vi "save ROI overlay for arbitrary line scan.vi"(11 "ROI Descriptor":T1 {"Contours"."Type" items=["No Selection", "Point", "Line", "Rectangle", "Oval", "Polygon", "Freehand Region", "Annulus", "Unused2", "Unused3", "Broken Line", "Freehand Line", "Rotated Rectangle"]}) -> ()   [LabVIEW 2017]
doc: "SciScan 1.2 160622"
uses:
  GFG/GFGImageRefsGet.vi
  GFG/GFGDisplayRefsGet.vi
  <vilib>/Utility/file.llb/Write To Spreadsheet File (I64).vi
  GFG/GFG library.lvlib
  <vilib>/vision/NI_Vision_Development_Module.lvlib
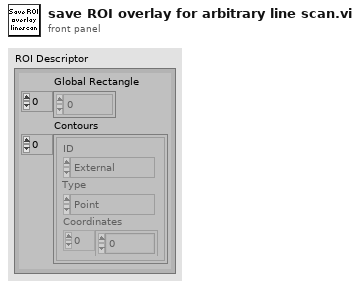
[diagram p1: front panel]
types:
  T1 = typedef "ROI Descriptor" = cluster{"Global Rectangle":i32[], "Contours":cluster{"ID":enum32{"External", "Internal"}, "Type":u32, "Coordinates":i32[]}[]}
  T2 = typedef "Image Type" = u32
  T3 = cluster{"Left":i32, "Top":i32, "Right":i32, "Bottom":i32}
  T4 = typedef "IMAQ Image.ctl" = refnum<image>
  T5 = cluster{"Channel 1 small":T4, "Channel 2 small":T4, "Channel 3 small":T4, "Channel 4 small":T4, "Channel 1 large":T4, "Channel 2 large":T4, "Channel 3 large":T4, "Channel 4 large":T4, "RGB overlay":T4, "ROI Image display":T4, "arb line scan display":T4, "Channel 5 large":T4}
  T6 = cluster{"Channel 1 small":refnum<vi>, "Channel 2 small":refnum<vi>, "Channel 3 small":refnum<vi>, "Channel 4 small":refnum<vi>, "Channel 1 large":refnum<vi>, "Channel 2 large":refnum<vi>, "Channel 3 large":refnum<vi>, "Channel 4 large":refnum<vi>, "RGB overlay":refnum<vi>, "ROI Image display":refnum<vi>, "arb line scan display":refnum<vi>, "Channel 5 large":refnum<vi>}
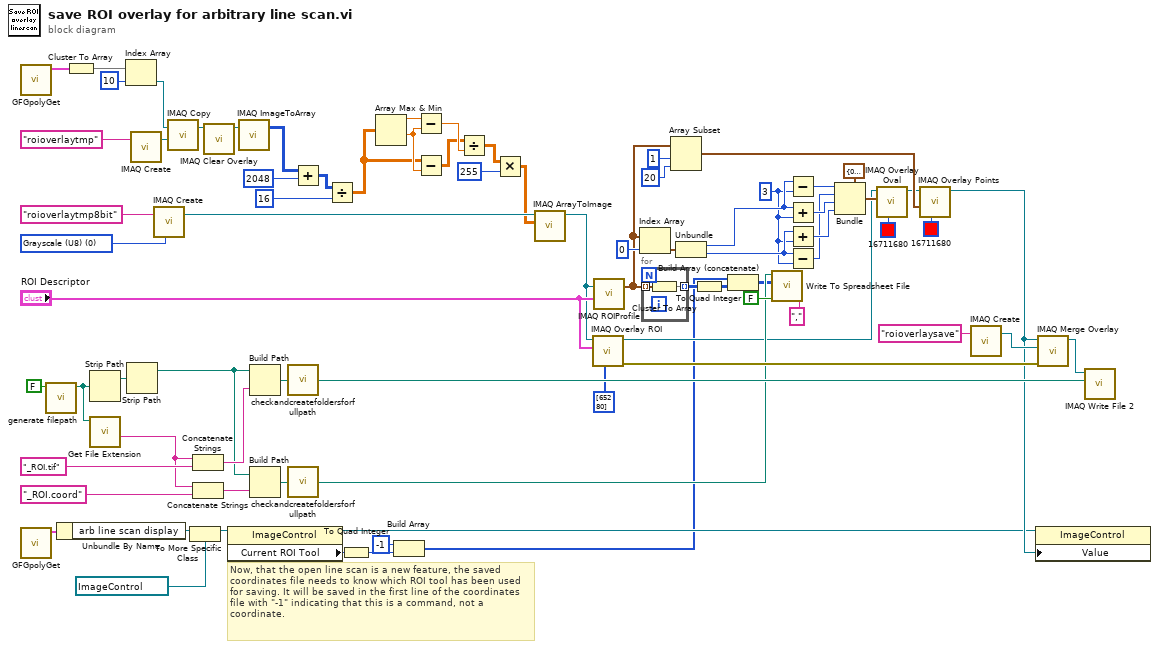
[diagram p0: block diagram]
diagram:
  w29 = T2 0 items=["Grayscale (U8)", "Grayscale (I16)", "Grayscale (SGL)", "Complex (CSG)", "RGB (U32)", "HSL (U32)", "RGB (U64)", "Grayscale (U16)"] ("Image Type")
  w11 = 3 ("y")
  # "Now, that the open line scan is a new feature, the saved coordinates file needs to know which ROI tool has been used for saving. It will be saved in the first line of the coordinates file with \"-1\" indicating that this is a command, not a coordinate."
  n1 = call-poly "GFGpolyGet.vi"() -> ("Image Refs Out"=w73:T5)  [unwired: 10 in, 1 out]
  n2 = call-poly "GFGpolyGet.vi"() -> ("DisplayRefsOut(generic class)"=w37:T6)  [unwired: 10 in, 1 out]
  n3 = call "generate filepath.vi"("set file.path GFG (default: T)"=FALSE) -> ("path"=w72:path)  [unwired: 10 in]
  n4 = Unbundle By Name(w37) -> ("arb line scan display"=w36:refnum<vi>)
  n5 = Cluster To Array(cluster=w73) -> (array=w75:T4[])
  n6 = Strip Path(path=w72) -> (stripped path=w68:path)  [unwired: 1 out]
  n7 = call <vilib>:"Get File Extension.vi"("file"=w72) -> ("filename without extension"=w63:string)  [unwired: 6 in, 4 out]
  n8 = Index Array(array=w75, index=10) -> (element=w23:T4)
  n9 = Strip Path(path=w68) -> (stripped path=w62:path)  [unwired: 1 out]
  n10 = call "IMAQ Create"("Image Name"="roioverlaytmp") -> ("New Image"=w33:T4)  [unwired: 4 in, 1 out]
  n11 = call "IMAQ Create"("Image Name"="roioverlaytmp8bit", "Image Type"=w29) -> ("New Image"=w24:T4)  [unwired: 3 in, 1 out]
  n12 = call "IMAQ Copy"("Image Dst"=w33, "Image Src"=w23) -> ("Image Dst Out"=w32:T4)  [unwired: 4 in, 1 out]
  n13 = To More Specific Class(target class=refnum<vi> refnum ("Image"), reference=w36) -> (specific class reference=w10:refnum<vi>)  [unwired: 1 in, 1 out]
  n14 = Concatenate Strings(w63, "_ROI.tif" ("string")) -> (w71:string)
  n15 = Concatenate Strings(w63, "_ROI.coord" ("string")) -> (w64:string)
  n16 = call "IMAQ Clear Overlay"("Image"=w32) -> ("Image Out"=w28:T4)  [unwired: 9 in, 1 out]
  n17 = property class="ImageControl"(reference=w10) -> (reference out=w9:refnum<vi>, "Current ROI Tool"=w6:u32)  [unwired: 1 in, 1 out]
  n18 = call "IMAQ ImageToArray"("Image"=w28) -> ("Image Pixels (I16)"=w22:i16[][])  [unwired: 3 in, 4 out]
  n19 = Build Path(base path=w62, name or relative path=w71) -> (appended path=w70:path)
  n20 = Build Path(base path=w62, name or relative path=w64) -> (appended path=w58:path)
  n21 = call "checkandcreatefoldersforfullpath.vi"("Path IN"=w70) -> ("Path OUT"=w69:path)  [unwired: 4 in]
  n22 = call "checkandcreatefoldersforfullpath.vi"("Path IN"=w58) -> ("Path OUT"=w57:path)  [unwired: 4 in]
  n23 = Add(x=w22, y=i16 2048 ("index")) -> (x+y=w26:i16[][])
  n24 = Divide(x=w26, y=i16 16 ("index")) -> (x/y=w18:dbl[][])
  n25 = To Quad Integer(1:w6) -> (0:w5:i64)
  n26 = Array Max & Min(array=w18) -> (max value=w20:dbl, min value=w19:dbl)  [unwired: 2 out]
  n27 = Build Array(i64 -1 ("element"), w5) -> (w4:i64[])
  n28 = Subtract(x=w20, y=w19) -> (x-y=w17:dbl)
  n29 = Subtract(x=w18, y=w19) -> (x-y=w16:dbl[][])
  n30 = Divide(x=w16, y=w17) -> (x/y=w15:dbl[][])
  n31 = Multiply(x=w15, y=i16 255 ("index")) -> (x*y=w14:dbl[][])
  n32 = call "IMAQ ArrayToImage"("Image Pixels (U8)"=w14, "Image"=w24) -> ("Image Out"=w21:T4)  [unwired: 8 in, 1 out]
  n33 = call "IMAQ Overlay ROI"("Colors (Green)"=u32[] [65280], "ROI Descriptor"="ROI Descriptor", "Image"=w21) -> ("error out"=w76:errorcluster, "Image Out"=w38:T4)  [unwired: 7 in]
  n34 = call "IMAQ ROIProfile"("ROI Descriptor"="ROI Descriptor", "Image"=w21) -> ("Pixel Coordinates"=w44:cluster{"X":u32, "Y":u32}[])  [unwired: 2 in, 4 out]
  n35 = Index Array(array=w44, index=0) -> (element=w53:cluster{"X":u32, "Y":u32})
  n36 = for {
    tunnel: w44 -> [w79] mode=indexing
    tunnel: [w78] -> w8 mode=indexing
    n37 = Cluster To Array(cluster=w79) -> (array=w78:u32[])
  }
  n38 = Array Subset(array=w44, index=1, length=20) -> (w41:cluster{"X":u32, "Y":u32}[])
  n39 = Unbundle(w53) -> ("X"=w47:u32, "Y"=w46:u32)
  n40 = To Quad Integer(1:w8) -> (0:w3:i64[][])
  n41 = Build Array (concatenate)(w4, w3) -> (w2:i64[][])
  n42 = call-poly <vilib>:"Write To Spreadsheet File.vi"("delimiter (\\t)"="," ("delimiter (\\t)"), "append to file? (new file:F)"=FALSE, "2D data"=w2, "file path (dialog if empty)"=w57) -> ()  [unwired: 4 in, 1 out]
  n43 = Subtract(x=w47, y=w11) -> (x-y=w51:u32)
  n44 = Add(x=w47, y=w11) -> (x+y=w52:u32)
  n45 = Add(x=w46, y=w11) -> (x+y=w50:u32)
  n46 = Subtract(x=w46, y=w11) -> (x-y=w49:u32)
  n47 = Bundle(cluster=T3 {"Left"=0, "Top"=0, "Right"=0, "Bottom"=0} ("Bounding Rectangle"), "Left"=w51, "Top"=w49, "Right"=w52, "Bottom"=w50) -> (w45:T3)
  n48 = call "IMAQ Overlay Oval"("Color"=u32 16711680, "Bounding Rectangle"=w45, "Image"=w38) -> ("Image Out"=w39:T4)  [unwired: 7 in, 1 out]
  n49 = call "IMAQ Overlay Points"("Color"=u32 16711680, "Array of Points"=w41, "Image"=w39) -> ("Image Out"=w31:T4)  [unwired: 7 in, 1 out]
  n50 = call "IMAQ Create"("Image Name"="roioverlaysave") -> ("New Image"=w60:T4)  [unwired: 4 in, 1 out]
  n51 = property class="ImageControl"(reference=w9, "Value"=w31) -> ()  [unwired: 1 in, 2 out]
  n52 = call "IMAQ Merge Overlay"("error in (no error)"=w76, "Image Dst"=w60, "Image Src"=w31) -> ("Image Dst Out"=w35:T4)  [unwired: 7 in, 1 out]
  n53 = call-poly "IMAQ Write File 2"("File Path"=w69, "Image"=w35) -> ()  [unwired: 8 in, 2 out]
